vi "Open Connection to All - Type Code Array - Ver 2.vi"(8 "Error In":errorcluster, 10 "Type Code":i32[](array[numeric]), 11 "URL":string[](array[string])) -> (0 "Error Out":errorcluster, 1 "Error Status":bool, 2 "Type Code":i32[](array[numeric]), 3 "Variable Refnum":variant[](array[variant]))   [LabVIEW 2014]
doc: "<B>Copyright</B>: (c) MHWirth 2015. All rights reserved.\n\nThis VI opens connection to all shared variables that are specified using URL and Type arrays. It converts the refnum to variant and send it out.\n\nIf the type is unknown (Error 7001) or read variable function is errorenous, the loop stops and Error Status is True. \n\n<B>Defined Types</B>:\nCode 1. Boolean\nCode 2 to 5. Int8/16/32/64\nCode 6 to 9. UInt8/16/32/64\nCode 10. Double\nCode 11. Single-precision\nCode 12. String\nCode 13 to 24. 1D array of xxx\nCode 25 to 36. 2D array of xxxs\n\n<B>Error 7001</B>: Unknown Data Type - Type Code Array (Int32) contains -1 indicating an unknown data type."
panel:
  out "no. deployed shared variables":i32
  out "Status":string
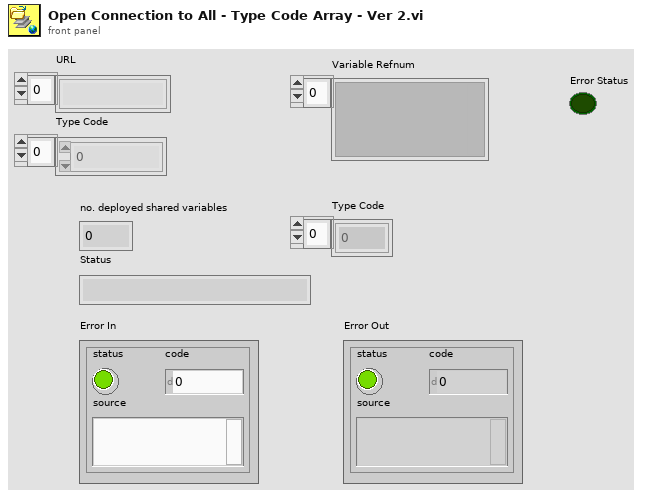
[diagram p1: front panel]
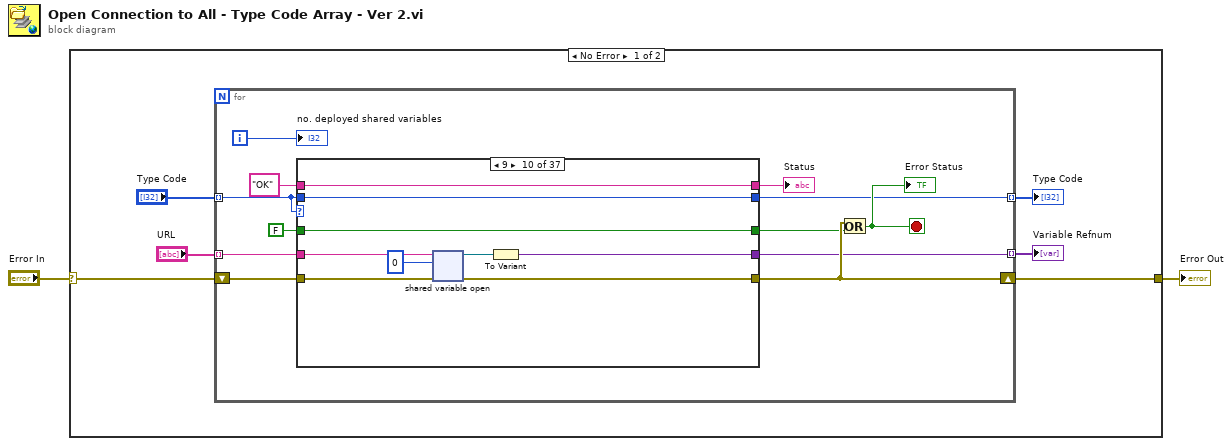
[diagram p0: block diagram]
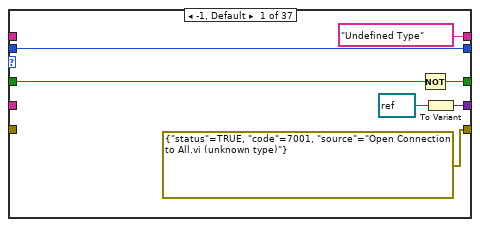
[diagram p2: hidden frame]
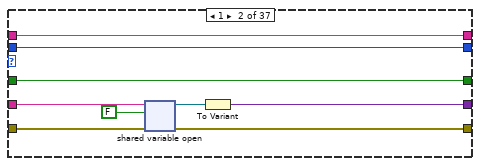
[diagram p3: hidden frame]
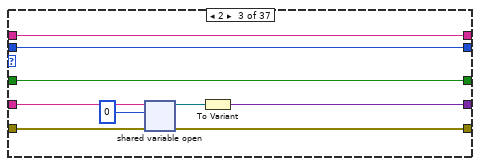
[diagram p4: hidden frame]
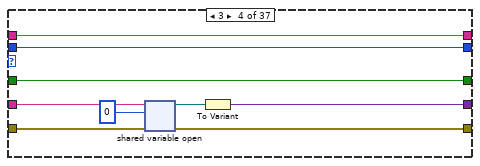
[diagram p5: hidden frame]
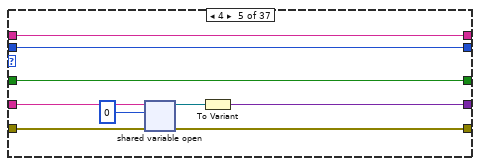
[diagram p6: hidden frame]
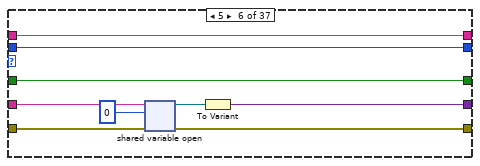
[diagram p7: hidden frame]
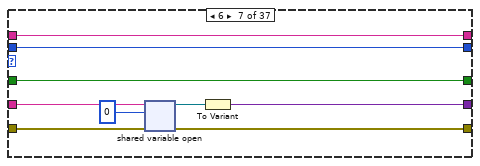
[diagram p8: hidden frame]
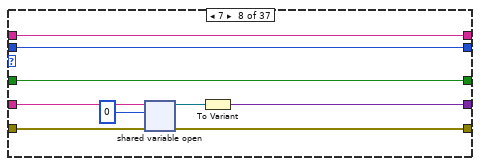
[diagram p9: hidden frame]
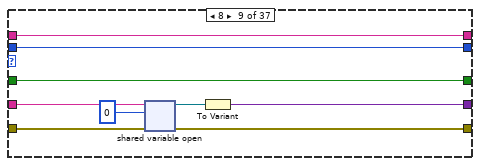
[diagram p10: hidden frame]
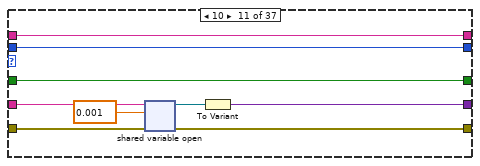
[diagram p11: hidden frame]
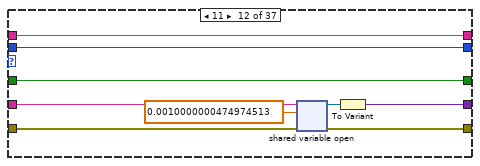
[diagram p12: hidden frame]
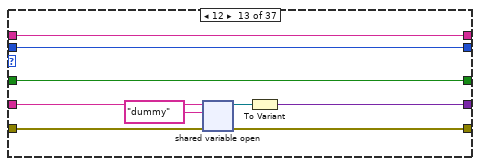
[diagram p13: hidden frame]
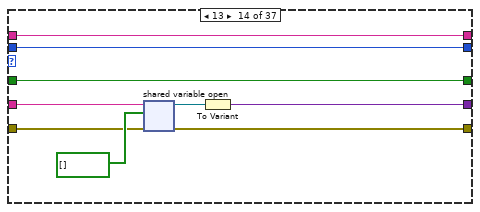
[diagram p14: hidden frame]
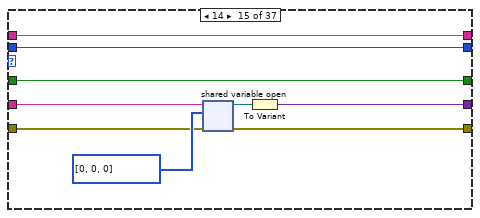
[diagram p15: hidden frame]
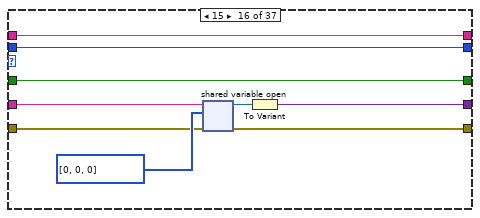
[diagram p16: hidden frame]
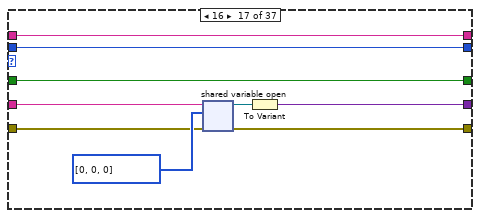
[diagram p17: hidden frame]
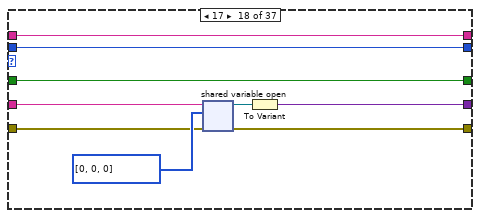
[diagram p18: hidden frame]
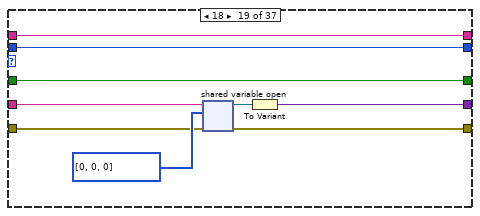
[diagram p19: hidden frame]
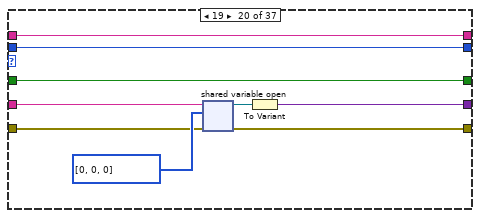
[diagram p20: hidden frame]
diagram:
  n1 = case shown="No Error" "Error In" {
    selector: "Error In" -> [w8 w352]
    tunnel: [w7 w352] -> w1
    frame No Error {
      n2 = for {
        tunnel: [w14] -> w4 mode=indexing
        shift-right: [w19] -> w7
        shift-left: w8 -> [w20]
        tunnel: "URL" -> [w13] mode=indexing
        tunnel: "Type Code" -> [w12] mode=indexing
        tunnel: [w9] -> w3 mode=indexing
        i -> [w10]
        stop <- w11 stop-if-true
        n3 = case shown="9" w12 {
          tunnel: w20 -> [_ w35 w44 w53 w62 w71 w80 w89 w98 w107 w116 w125 w135 w143 w152 w161 w170 w179 w188 w197 w206 w215 w224 w233 w242 w251 w260 w269 w278 w287 w296 w305 w314 w323 w332 w341 w350]
          tunnel: [errorcluster {"status"=TRUE, "code"=7001, "source"="Open Connection to All.vi (unknown type)"} ("error constant") w32 w41 w50 w59 w68 w77 w86 w95 w104 w113 w122 w131 w140 w149 w158 w167 w176 w185 w194 w203 w212 w220 w230 w239 w248 w257 w266 w275 w284 w293 w302 w311 w320 w329 w338 w347] -> w19
          tunnel: ["Undefined Type" w34 w43 w52 w61 w70 w79 w88 w97 w106 w115 w124 w134 w142 w151 w160 w169 w178 w187 w196 w205 w214 w223 w232 w241 w250 w259 w268 w277 w286 w295 w304 w313 w322 w331 w340 w349] -> w18
          tunnel: "OK" -> [_ w34 w43 w52 w61 w70 w79 w88 w97 w106 w115 w124 w134 w142 w151 w160 w169 w178 w187 w196 w205 w214 w223 w232 w241 w250 w259 w268 w277 w286 w295 w304 w313 w322 w331 w340 w349]
          tunnel: FALSE -> [w26 w33 w42 w51 w60 w69 w78 w87 w96 w105 w114 w123 w133 w141 w150 w159 w168 w177 w186 w195 w204 w213 w222 w231 w240 w249 w258 w267 w276 w285 w294 w303 w312 w321 w330 w339 w348]
          tunnel: [w25 w33 w42 w51 w60 w69 w78 w87 w96 w105 w114 w123 w133 w141 w150 w159 w168 w177 w186 w195 w204 w213 w222 w231 w240 w249 w258 w267 w276 w285 w294 w303 w312 w321 w330 w339 w348] -> w15
          tunnel: w13 -> [_ w31 w40 w49 w58 w67 w76 w85 w94 w103 w112 w121 w130 w139 w148 w157 w166 w175 w184 w193 w202 w211 w221 w229 w238 w247 w256 w265 w274 w283 w292 w301 w310 w319 w328 w337 w346]
          tunnel: [w22 w29 w38 w47 w56 w65 w74 w83 w92 w101 w110 w119 w128 w137 w146 w155 w164 w173 w182 w191 w200 w209 w218 w227 w236 w244 w253 w262 w271 w280 w289 w298 w307 w316 w325 w334 w343] -> w14
          tunnel: w12 -> [w21 w28 w37 w46 w55 w64 w73 w82 w91 w100 w109 w118 w127 w136 w145 w154 w163 w172 w181 w190 w199 w208 w217 w226 w235 w246 w255 w264 w273 w282 w291 w300 w309 w318 w327 w336 w345]
          tunnel: [w21 w28 w37 w46 w55 w64 w73 w82 w91 w100 w109 w118 w127 w136 w145 w154 w163 w172 w181 w190 w199 w208 w217 w226 w235 w246 w255 w264 w273 w282 w291 w300 w309 w318 w327 w336 w345] -> w9
          frame -1, Default {
            n4 = Not(x=w26) -> (.not. x?=w25:bool)
            n5 = To Variant(anything=refnum<k21> refnum) -> (Variant=w22:variant)
          }
          frame 1 {
            n6 = shared-variable-open(w31, w35, FALSE) -> (w30:refnum<k21>, w32:errorcluster)  [unwired: 1 in]
            n7 = To Variant(anything=w30) -> (Variant=w29:variant)
          }
          frame 2 {
            n8 = shared-variable-open(w40, w44, i8 0) -> (w39:refnum<k21>, w41:errorcluster)  [unwired: 1 in]
            n9 = To Variant(anything=w39) -> (Variant=w38:variant)
          }
          frame 3 {
            n10 = shared-variable-open(w49, w53, i16 0) -> (w48:refnum<k21>, w50:errorcluster)  [unwired: 1 in]
            n11 = To Variant(anything=w48) -> (Variant=w47:variant)
          }
          frame 4 {
            n12 = shared-variable-open(w58, w62, 0) -> (w57:refnum<k21>, w59:errorcluster)  [unwired: 1 in]
            n13 = To Variant(anything=w57) -> (Variant=w56:variant)
          }
          frame 5 {
            n14 = shared-variable-open(w67, w71, i64 0) -> (w66:refnum<k21>, w68:errorcluster)  [unwired: 1 in]
            n15 = To Variant(anything=w66) -> (Variant=w65:variant)
          }
          frame 6 {
            n16 = shared-variable-open(w76, w80, u8 0) -> (w75:refnum<k21>, w77:errorcluster)  [unwired: 1 in]
            n17 = To Variant(anything=w75) -> (Variant=w74:variant)
          }
          frame 7 {
            n18 = shared-variable-open(w85, w89, u16 0) -> (w84:refnum<k21>, w86:errorcluster)  [unwired: 1 in]
            n19 = To Variant(anything=w84) -> (Variant=w83:variant)
          }
          frame 8 {
            n20 = shared-variable-open(w94, w98, u32 0) -> (w93:refnum<k21>, w95:errorcluster)  [unwired: 1 in]
            n21 = To Variant(anything=w93) -> (Variant=w92:variant)
          }
          frame 9 {
            n22 = shared-variable-open(w103, w107, u64 0) -> (w102:refnum<k21>, w104:errorcluster)  [unwired: 1 in]
            n23 = To Variant(anything=w102) -> (Variant=w101:variant)
          }
          frame 10 {
            n24 = shared-variable-open(w112, w116, 0.001) -> (w111:refnum<k21>, w113:errorcluster)  [unwired: 1 in]
            n25 = To Variant(anything=w111) -> (Variant=w110:variant)
          }
          frame 11 {
            n26 = shared-variable-open(w121, w125, sgl 0.001) -> (w120:refnum<k21>, w122:errorcluster)  [unwired: 1 in]
            n27 = To Variant(anything=w120) -> (Variant=w119:variant)
          }
          frame 12 {
            n28 = shared-variable-open(w130, w135, "dummy") -> (w129:refnum<k21>, w131:errorcluster)  [unwired: 1 in]
            n29 = To Variant(anything=w129) -> (Variant=w128:variant)
          }
          frame 13 {
            n30 = shared-variable-open(w139, w143, bool[] []) -> (w138:refnum<k21>, w140:errorcluster)  [unwired: 1 in]
            n31 = To Variant(anything=w138) -> (Variant=w137:variant)
          }
          frame 14 {
            n32 = shared-variable-open(w148, w152, i8[] [0, 0, 0]) -> (w147:refnum<k21>, w149:errorcluster)  [unwired: 1 in]
            n33 = To Variant(anything=w147) -> (Variant=w146:variant)
          }
          frame 15 {
            n34 = shared-variable-open(w157, w161, i16[] [0, 0, 0]) -> (w156:refnum<k21>, w158:errorcluster)  [unwired: 1 in]
            n35 = To Variant(anything=w156) -> (Variant=w155:variant)
          }
          frame 16 {
            n36 = shared-variable-open(w166, w170, i32[] [0, 0, 0]) -> (w165:refnum<k21>, w167:errorcluster)  [unwired: 1 in]
            n37 = To Variant(anything=w165) -> (Variant=w164:variant)
          }
          frame 17 {
            n38 = shared-variable-open(w175, w179, i64[] [0, 0, 0]) -> (w174:refnum<k21>, w176:errorcluster)  [unwired: 1 in]
            n39 = To Variant(anything=w174) -> (Variant=w173:variant)
          }
          frame 18 {
            n40 = shared-variable-open(w184, w188, u8[] [0, 0, 0]) -> (w183:refnum<k21>, w185:errorcluster)  [unwired: 1 in]
            n41 = To Variant(anything=w183) -> (Variant=w182:variant)
          }
          frame 19 {
            n42 = shared-variable-open(w193, w197, u16[] [0, 0, 0]) -> (w192:refnum<k21>, w194:errorcluster)  [unwired: 1 in]
            n43 = To Variant(anything=w192) -> (Variant=w191:variant)
          }
          frame 20 {
            n44 = shared-variable-open(w202, w206, u32[] [0, 0, 0]) -> (w201:refnum<k21>, w203:errorcluster)  [unwired: 1 in]
            n45 = To Variant(anything=w201) -> (Variant=w200:variant)
          }
          frame 21 {
            n46 = shared-variable-open(w211, w215, u64[] [0, 0, 0]) -> (w210:refnum<k21>, w212:errorcluster)  [unwired: 1 in]
            n47 = To Variant(anything=w210) -> (Variant=w209:variant)
          }
          frame 22 {
            n48 = shared-variable-open(w221, w224, dbl[] [0.0, 0.0, 0.0]) -> (w219:refnum<k21>, w220:errorcluster)  [unwired: 1 in]
            n49 = To Variant(anything=w219) -> (Variant=w218:variant)
          }
          frame 23 {
            n50 = shared-variable-open(w229, w233, sgl[] [0.0, 0.0, 0.0]) -> (w228:refnum<k21>, w230:errorcluster)  [unwired: 1 in]
            n51 = To Variant(anything=w228) -> (Variant=w227:variant)
          }
          frame 24 {
            n52 = shared-variable-open(w238, w242, string[] []) -> (w237:refnum<k21>, w239:errorcluster)  [unwired: 1 in]
            n53 = To Variant(anything=w237) -> (Variant=w236:variant)
          }
          frame 25 {
            n54 = shared-variable-open(w247, w251, bool[][] []) -> (w245:refnum<k21>, w248:errorcluster)  [unwired: 1 in]
            n55 = To Variant(anything=w245) -> (Variant=w244:variant)
          }
          frame 26 {
            n56 = shared-variable-open(w256, w260, i8[][] [[0, 0, 0]]) -> (w254:refnum<k21>, w257:errorcluster)  [unwired: 1 in]
            n57 = To Variant(anything=w254) -> (Variant=w253:variant)
          }
          frame 27 {
            n58 = shared-variable-open(w265, w269, i16[][] [[0, 0, 0]]) -> (w263:refnum<k21>, w266:errorcluster)  [unwired: 1 in]
            n59 = To Variant(anything=w263) -> (Variant=w262:variant)
          }
          frame 28 {
            n60 = shared-variable-open(w274, w278, i32[][] [[0, 0, 0]]) -> (w272:refnum<k21>, w275:errorcluster)  [unwired: 1 in]
            n61 = To Variant(anything=w272) -> (Variant=w271:variant)
          }
          frame 29 {
            n62 = shared-variable-open(w283, w287, i64[][] [[0, 0, 0]]) -> (w281:refnum<k21>, w284:errorcluster)  [unwired: 1 in]
            n63 = To Variant(anything=w281) -> (Variant=w280:variant)
          }
          frame 30 {
            n64 = shared-variable-open(w292, w296, u8[][] [[0, 0, 0]]) -> (w290:refnum<k21>, w293:errorcluster)  [unwired: 1 in]
            n65 = To Variant(anything=w290) -> (Variant=w289:variant)
          }
          frame 31 {
            n66 = shared-variable-open(w301, w305, u16[][] [[0, 0, 0]]) -> (w299:refnum<k21>, w302:errorcluster)  [unwired: 1 in]
            n67 = To Variant(anything=w299) -> (Variant=w298:variant)
          }
          frame 32 {
            n68 = shared-variable-open(w310, w314, u32[][] [[0, 0, 0]]) -> (w308:refnum<k21>, w311:errorcluster)  [unwired: 1 in]
            n69 = To Variant(anything=w308) -> (Variant=w307:variant)
          }
          frame 33 {
            n70 = shared-variable-open(w319, w323, u64[][] [[0, 0, 0]]) -> (w317:refnum<k21>, w320:errorcluster)  [unwired: 1 in]
            n71 = To Variant(anything=w317) -> (Variant=w316:variant)
          }
          frame 34 {
            n72 = shared-variable-open(w328, w332, dbl[][] [[0.0, 0.0, 0.0]]) -> (w326:refnum<k21>, w329:errorcluster)  [unwired: 1 in]
            n73 = To Variant(anything=w326) -> (Variant=w325:variant)
          }
          frame 35 {
            n74 = shared-variable-open(w337, w341, sgl[][] [[0.0, 0.0, 0.0]]) -> (w335:refnum<k21>, w338:errorcluster)  [unwired: 1 in]
            n75 = To Variant(anything=w335) -> (Variant=w334:variant)
          }
          frame 36 {
            n76 = shared-variable-open(w346, w350, string[][] []) -> (w344:refnum<k21>, w347:errorcluster)  [unwired: 1 in]
            n77 = To Variant(anything=w344) -> (Variant=w343:variant)
          }
        }
        "Status" <- w18
        n78 = Or(x=w19, y=w15) -> (x .or. y?=w11:bool)
        "Error Status" <- w11
        "no. deployed shared variables" <- w10
      }
      "Variable Refnum" <- w4
      "Type Code" <- w3
    }
    frame Error {
    }
  }
  "Error Out" <- w1
